vi "Set processing data API.vi"(8 "Error In":errorcluster, 10 "Waveform name":string, 11 "Waveform":waveform(dbl)) -> (0 "Error Out":errorcluster)   [LabVIEW 2017, in "UI.lvlib"]
uses:
  UI.lvlib
  Controls/Command Data [cluster].ctl
  Controls/Commands [enum].ctl
  Events/Events.lvlib
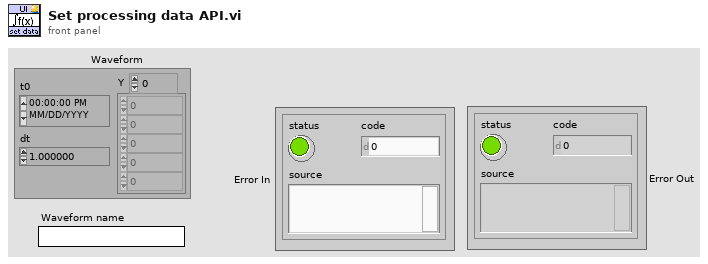
[diagram p1: front panel]
types:
  T1 = typedef "UI.lvlib/Command Data [cluster].ctl" = cluster{"Command":T2, "Data":variant}
  T2 = typedef "UI.lvlib/Commands [enum].ctl" = enum16{"Start", "Update", "Acquisition Complete", "Stop", "Set DAQ data", "Set Scope data", "Set processing data", "Clear Graphs"}
  T3 = cluster{"Waveform":waveform(dbl), "Waveform name":string}
  T4 = typedef "Events.lvlib/Refs [cluster].ctl" = cluster{"Exit":refnum<user-event>, "Controller":refnum<user-event>, "System Error":refnum<user-event>, "UI":refnum<user-event>, "Example Module":refnum<user-event>, "Shutter":refnum<user-event>, "Monochromator":refnum<user-event>, "DAQ":refnum<user-event>, "Scope":refnum<user-event>, "Processing":refnum<user-event>, "File IO":refnum<user-event>, "Colour wheel":refnum<user-event>}
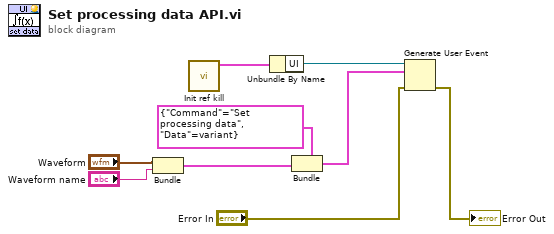
[diagram p0: block diagram]
diagram:
  n1 = Bundle("Waveform"="Waveform", "Waveform name"="Waveform name") -> (w1:T3)  [unwired: 1 in]
  n2 = call "Init ref kill.vi"() -> ("Messages"=w9:T4)  [unwired: 10 in, 1 out]
  n3 = Unbundle By Name(w9) -> ("UI"=w8:refnum<user-event>)
  n4 = Bundle(cluster=T1 {"Command"=enum."Set processing data", "Data"=variant} ("event data"), "Data"=w1) -> (w4:T1)  [unwired: 1 in]
  n5 = Generate User Event(user event=w8, event data cluster=w4, error in="Error In") -> (error out=→"Error Out":errorcluster)  [unwired: 1 in, 1 out]
